vi "wavecgi.vi"   [LabVIEW 2012]
uses:
  <vilib>/addons/internet/NI_InternetTK_Core_VIs.lvlib
types:
  T1 = typedef "CGI Connection Info.ctl" = cluster{"name":string, "type":T2, "session":T3}
  T2 = typedef "CGI Request Type.ctl" = enum16{"cgi", ".spool first", ".spool", ".spool last"}
  T3 = typedef "HTTP Session.ctl" = refnum<k1>
  T4 = typedef "NI_FTP.lvlib/Keyed Array.ctl" = cluster{"keys":string[], "values":string[]}
  T5 = typedef "Wave CGI PArams.ctl" = cluster{"low":string, "high":string, "steps":string, "form":string, "target":string, "spool":string}
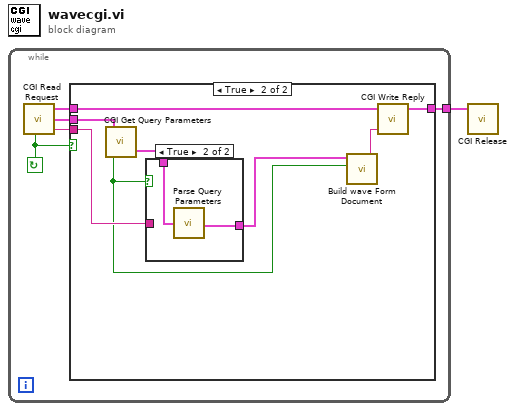
[diagram p0: block diagram]
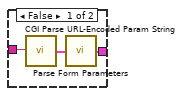
[diagram p3: hidden frame]
diagram:
  n1 = while {
    tunnel: [w5] -> w1
    stop <- w4 continue-if-true
    n2 = call <vilib>:"CGI Read Request.vi"() -> ("valid request?"=w4:bool, "cgi connection info"=w6:T1, "env"=w3:T4, "content"=w2:string)  [unwired: 4 in]
    n3 = case shown="True" w4 {
      tunnel: [w7 w15] -> w5
      tunnel: w6 -> [w7 w14]
      tunnel: w3 -> [_ w13]
      tunnel: w2 -> [_ w12]
      frame False {
      }
      frame True {
        n4 = call <vilib>:"CGI Get Query Parameters.vi"("env"=w13) -> ("query params"=w11:T4, "has query string"=w8:bool)  [unwired: 1 out]
        n5 = case shown="True" w8 {
          tunnel: w12 -> [w18 _]
          tunnel: w11 -> [_ w20]
          tunnel: [w16 w19] -> w9
          frame False {
            n6 = call <vilib>:"CGI Parse URL-Encoded Param String.vi"("url-encoded param string"=w18) -> ("params"=w17:T4)
            n7 = call "Parse Form Parameters.vi"("form params"=w17) -> ("params"=w16:T5)
          }
          frame True {
            n8 = call "Parse Query Parameters.vi"("query params"=w20) -> ("params"=w19:T5)
          }
        }
        n9 = call "Build wave Form Document.vi"("form only? (F)"=w8, "params"=w9) -> ("form"=w10:string)  [unwired: 5 in]
        n10 = call <vilib>:"CGI Write Reply.vi"("content"=w10, "cgi connection info"=w14) -> ("cgi connection info out"=w15:T1)  [unwired: 3 in]
      }
    }
  }
  n11 = call <vilib>:"CGI Release.vi"("cgi connection info"=w1) -> ()  [unwired: 5 in]
